vi "RegisterNBitSwitchFull.vi"(5 "Switch Bit":bool=TRUE, 8 "error in":errorcluster, 9 "IP":string="172.16.17.47", 11 "Port":u16=9764) -> (0 "error out":errorcluster)   [LabVIEW 2012]
panel:
  in  "Device":u16(ring) items=["Attenuation", "Clipping", "Enable channel", "Delay line", "ASIC", "Enable L1 ch", "ASIC L1"]
  in  "N Bit":u16=10
  in  "Register Number":u16=4
  out "Register Swapped":u32=1078
  out "Register swap":dbl[](array[numeric])=[0.0, 1.0, 1.0, 0.0, 1.0, 1.0, 0.0, 0.0, 0.0, 0.0, 1.0, 0.0, 0.0, 0.0, 0.0, 0.0, 0.0, 0.0, 0.0, 0.0, 0.0, 0.0, 0.0, 0.0, 0.0, 0.0, 0.0, 0.0, 0.0, 0.0, 0.0, 0.0]
  out "Register Read":dbl[](array[numeric])=[0.0, 1.0, 1.0, 0.0, 1.0, 1.0, 0.0, 0.0, 0.0, 0.0, 1.0, 0.0, 0.0, 0.0, 0.0, 0.0, 0.0, 0.0, 0.0, 0.0, 0.0, 0.0, 0.0, 0.0, 0.0, 0.0, 0.0, 0.0, 0.0, 0.0, 0.0, 0.0]
  out "Register read":u32=1078
  # "0     1     2     3     4    5     6     7     8    9    10   11  12   13   14   15"
  # "0     1     2     3     4    5     6     7     8    9    10   11  12   13   14   15"
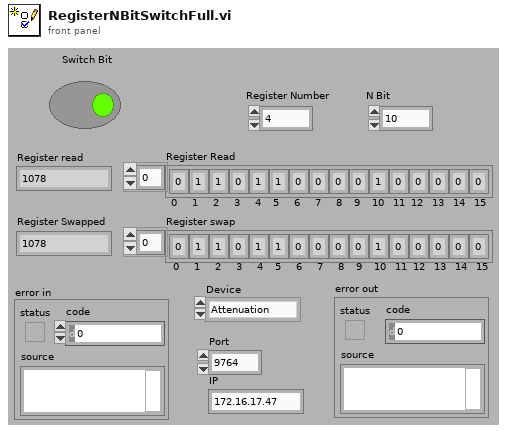
[diagram p1: front panel]
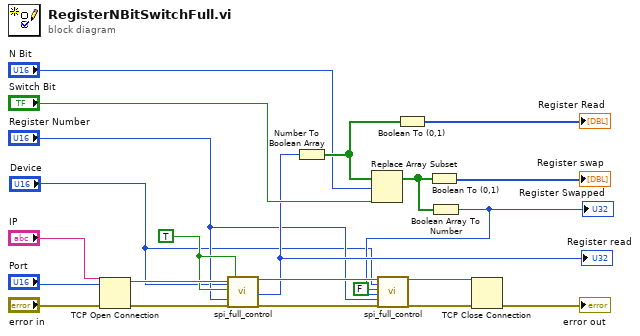
[diagram p0: block diagram]
diagram:
  w7 = TRUE
  n1 = TCP Open Connection(address="IP", remote port or service name="Port", error in (no error)="error in") -> (connection ID=w19:refnum<k5>, error out=w20:errorcluster)  [unwired: 2 in]
  n2 = call "spi_full_control.vi"("connection ID"=w19, "Device"="Device", "Read/#write"=w7, "Register or channel"="Register Number", "error out 3"=w20, "Read physical"=w7) -> ("connection ID out"=w9:refnum<k5>, "data read value"=w6:u32, "error out 2"=w10:errorcluster)  [unwired: 6 in, 5 out]
  "Register read" <- w6
  n3 = Number To Boolean Array(number=w6) -> (Boolean array=w15:bool[])
  n4 = Replace Array Subset(array=w15, new element="Switch Bit", index="N Bit") -> (w12:bool[])
  n5 = Boolean To (0,1)(Boolean=w15) -> (0, 1=→"Register Read":i16[])
  n6 = Boolean To (0,1)(Boolean=w12) -> (0, 1=→"Register swap":i16[])
  n7 = Boolean Array To Number(Boolean array=w12) -> (number=w3:u32)
  "Register Swapped" <- w3
  n8 = call "spi_full_control.vi"("connection ID"=w9, "Device"="Device", "Read/#write"=FALSE, "Data"=w3, "Register or channel"="Register Number", "error out 3"=w10) -> ("connection ID out"=w8:refnum<k5>, "error out 2"=w11:errorcluster)  [unwired: 6 in, 6 out]
  n9 = TCP Close Connection(connection ID=w8, error in (no error)=w11) -> (error out=→"error out":errorcluster)  [unwired: 1 in, 1 out]
